vi "test_libssh2_channel_free.vi"() -> ()   [LabVIEW 2017, in "integration_tests.lvlib"]
uses:
  integration_tests.lvlib
  libssh2/libssh2_channel_open_ex.vi
  support/support.lvlib
  libssh2/libssh2.lvlib
  <vilib>/PNR/Transparent Assertions/Transparent Assertions/Transparent Assertions.lvlib
panel:
  out "error out":errorcluster
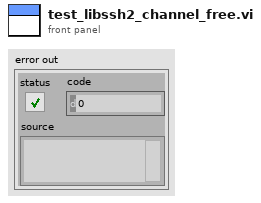
[diagram p1: front panel]
types:
  T1 = typedef "libssh2.lvlib/Session Refnum.ctl" = refnum<k1>
  T2 = typedef "libssh2.lvlib/Channel Refnum.ctl" = refnum<k1>
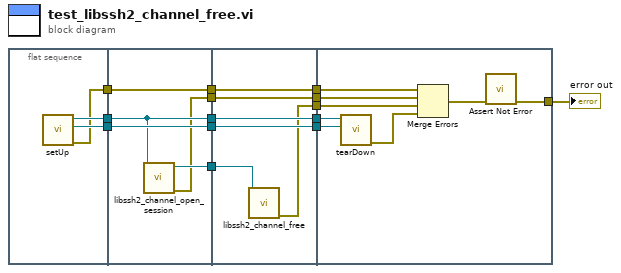
[diagram p0: block diagram]
diagram:
  n1 = flat-sequence {
    tunnel: [w17] -> w14
    tunnel: [w16] -> w13
    tunnel: [w15] -> w8
    tunnel: w14 -> [w21]
    tunnel: w13 -> [w22]
    tunnel: [w21] -> w6
    tunnel: [w22] -> w5
    tunnel: [w20] -> w4
    tunnel: w8 -> [w19]
    tunnel: [w19] -> w3
    tunnel: [w18] -> w2
    tunnel: w6 -> [w28]
    tunnel: w5 -> [w27]
    tunnel: w4 -> [w26]
    tunnel: [w28] -> w12
    tunnel: [w27] -> w11
    tunnel: [w25] -> w9
    tunnel: w3 -> [w24]
    tunnel: [w24] -> w7
    tunnel: w2 -> [w25]
    tunnel: [w23] -> w1
    tunnel: w12 -> [w36]
    tunnel: w11 -> [w35]
    tunnel: [w34] -> w10
    tunnel: w9 -> [w32]
    tunnel: w7 -> [w31]
    tunnel: w1 -> [w29]
    frame #0 {
      n2 = call "setUp.vi"() -> ("error out"=w15:errorcluster, "connection ID"=w16:refnum<k5>, "session"=w17:T1)  [unwired: 9 in]
    }
    frame #1 {
      n3 = call "libssh2_channel_open_session.vi"("session"=w21) -> ("error out"=w18:errorcluster, "channel"=w20:T2)  [unwired: 9 in]
    }
    frame #2 {
      n4 = call "libssh2_channel_free.vi"("channel"=w26) -> ("error out"=w23:errorcluster)  [unwired: 10 in]
    }
    frame #3 {
      n5 = call "tearDown.vi"("connection ID"=w35, "session"=w36) -> ("error out"=w33:errorcluster)  [unwired: 9 in]
      n6 = Merge Errors(w31, w32, w29, w33) -> (w30:errorcluster)
      n7 = call <vilib>:"Assert Not Error.vi"("error in (no error)"=w30) -> ("error out"=w34:errorcluster)  [unwired: 10 in]
    }
  }
  "error out" <- w10
